vi "Set Active User Machine Input.vi"() -> (3 "Machine Out":string)   [LabVIEW 2016]
uses:
  <userlib>/_MGI/Application Control/MGI VI Reference/MGI Current VI's Reference.vi
panel:
  in  "OK Button":bool
  in  "Which machine are you using?":string(combo)
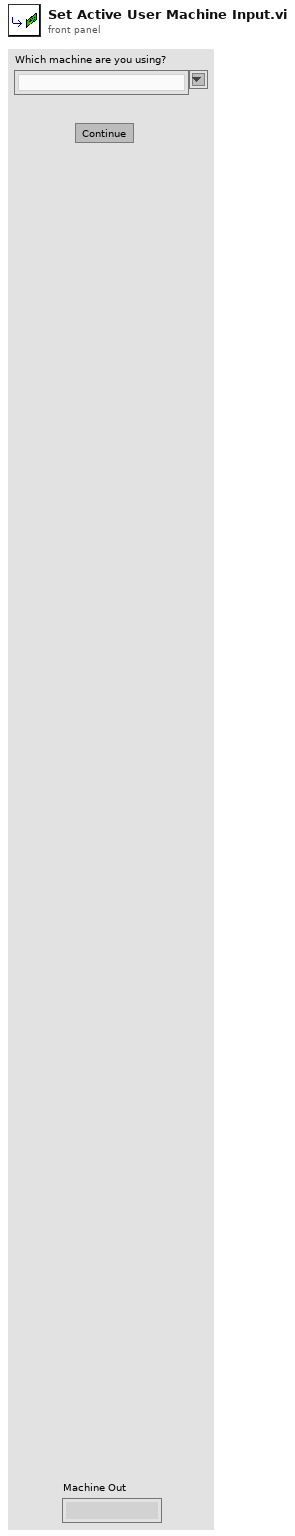
[diagram p1: front panel]
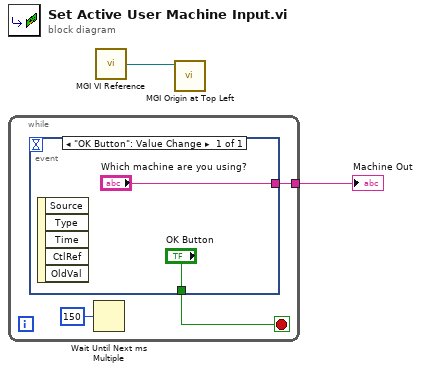
[diagram p0: block diagram]
diagram:
  n1 = while {
    tunnel: [w5] -> w2
    stop <- w4 stop-if-true
    n2 = event shown="[0] \"OK Button\": Value Change" {
      selector: _ -> [_]
      dyn-events: _ -> [_]
      timeout: _ -> [_]
      tunnel: ["Which machine are you using?"] -> w5
      tunnel: ["OK Button"] -> w4
      event "OK Button": Value Change {
        n3 = event-data() -> ()  [unwired: 1 in, 5 out]
      }
    }
    n4 = Wait Until Next ms Multiple(millisecond multiple=u32 150) -> ()  [unwired: 1 out]
  }
  "Machine Out" <- w2
  n5 = call-poly <userlib>:"MGI VI Reference.vi"() -> ("Current VI's Reference"=w1:refnum<vi>)  [unwired: 1 in]
  n6 = call <userlib>:"MGI Origin at Top Left.vi"("VI Reference In (Caller)"=w1) -> ()  [unwired: 8 in, 2 out]
